vi "SetStartingPointAndLocations.vi"(8 "error in (no error)":errorcluster, 9 "locations":T1[](array[typedef]), 10 "point":T1, 11 "PathTree in":refnum<class "RouteTree.lvclass">) -> (0 "error out":errorcluster, 3 "PathTree out":refnum<class "RouteTree.lvclass">)   [LabVIEW 2009, in "RouteTree.lvclass"]
uses:
  RouteTree.lvclass
  Waypoint/point.ctl
  Waypoint/Waypoint.lvclass
  Tree/Tree.lvclass
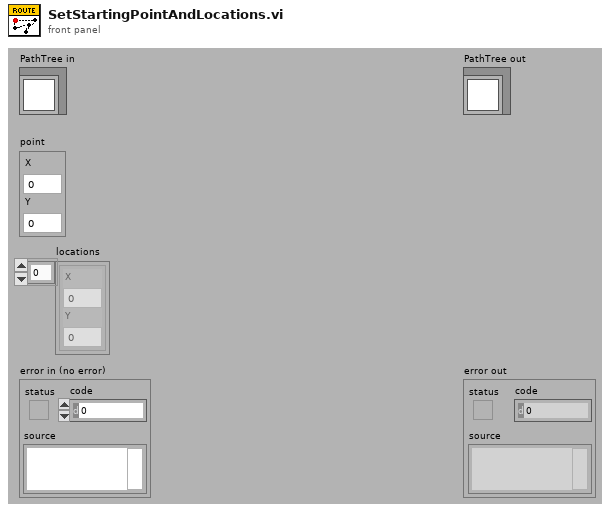
[diagram p1: front panel]
types:
  T1 = typedef "Waypoint.lvclass/point.ctl" = cluster{"X":dbl, "Y":dbl}
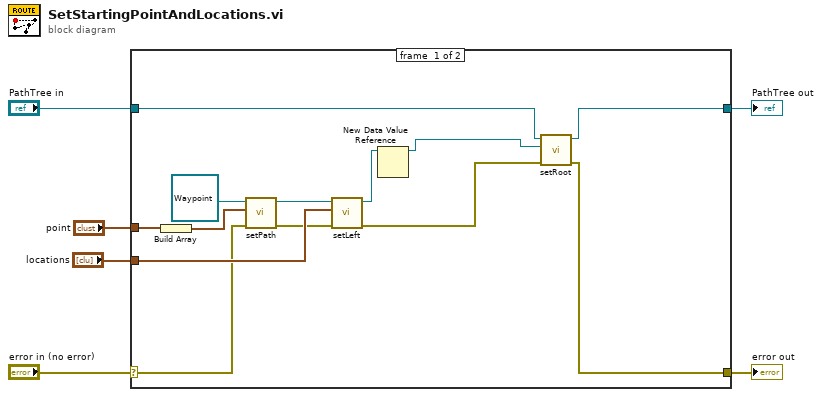
[diagram p0: block diagram]
diagram:
  n1 = case shown="No Error" "error in (no error)" {
    selector: "error in (no error)" -> [w12 w21]
    tunnel: [w16 w21] -> w5
    tunnel: [w17 w20] -> w3
    tunnel: "PathTree in" -> [w18 w20]
    tunnel: "point" -> [w11 _]
    tunnel: "locations" -> [w19 _]
    frame #0 {
      n2 = Build Array(w11) -> (w10:T1[])
      n3 = call "setPath.vi"("error in (no error)"=w12, "Path"=w10, "Waypoint in"=refnum<class "Waypoint.lvclass"> refnum ("Waypoint.lvclass")) -> ("error out"=w13:errorcluster, "Waypoint out"=w15:refnum<class "Waypoint.lvclass">)  [unwired: 7 in]
      n4 = call "setLeft.vi"("error in (no error)"=w13, "left"=w19, "Waypoint in"=w15) -> ("error out"=w7:errorcluster, "Waypoint out"=w9:refnum<class "Waypoint.lvclass">)  [unwired: 7 in]
      n5 = New Data Value Reference(data value=w9) -> (data value reference=w8:refnum<data-value>)  [unwired: 1 in, 1 out]
      n6 = call "setRoot.vi"("error in (no error)"=w7, "Root"=w8, "Tree in"=w18) -> ("error out"=w16:errorcluster, "Tree out"=w17:refnum<class "RouteTree.lvclass">)  [unwired: 7 in]
    }
    frame #1 {
    }
  }
  "error out" <- w5
  "PathTree out" <- w3
